vi "cluster error.vi"() -> ()   [LabVIEW 2016]
panel:
  out "Triangle 2":dynamicdata(graph) caption="Triangle"
  out "Sine 2":dynamicdata(graph) caption="Sine"
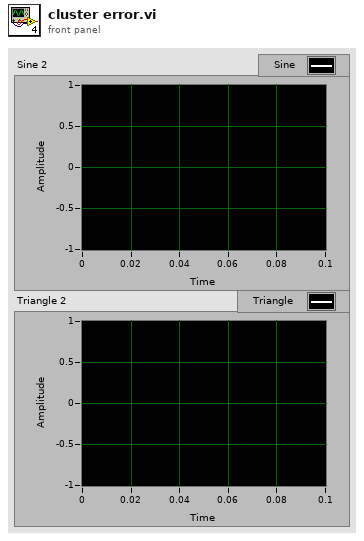
[diagram p1: front panel]
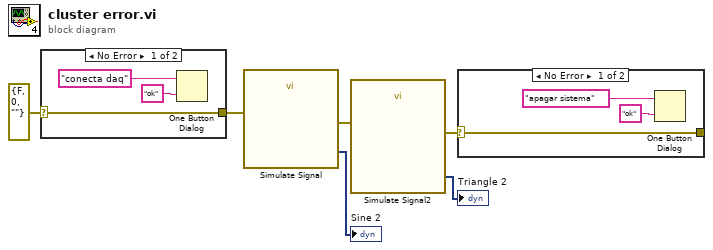
[diagram p0: block diagram]
diagram:
  n1 = case shown="No Error" errorcluster {"status"=FALSE, "code"=0, "source"=""} ("error constant") {
    selector: errorcluster {"status"=FALSE, "code"=0, "source"=""} ("error constant") -> [w9 w10]
    tunnel: [w9 w10] -> w3
    frame No Error {
      n2 = One Button Dialog(message="conecta daq", button name ("OK")="ok") -> ()  [unwired: 1 out]
    }
    frame Error {
    }
  }
  n3 = call "Simulate Signal"("error in (no error)"=w3) -> ("Sine"=→"Sine 2":dynamicdata, "error out"=w2:errorcluster)  [unwired: 13 in]
  n4 = call "Simulate Signal2"("error in (no error)"=w2) -> ("Triangle"=→"Triangle 2":dynamicdata, "error out"=w1:errorcluster)  [unwired: 13 in]
  n5 = case shown="No Error" w1 {
    selector: w1 -> [w11 w14]
    tunnel: [w11 w14] -> _
    frame No Error {
      n6 = One Button Dialog(message="apagar sistema", button name ("OK")="ok") -> ()  [unwired: 1 out]
    }
    frame Error {
    }
  }
